vi "Start.vi"(8 "error in":errorcluster, 10 "ASync [T]":bool, 11 "ServiceBase out":refnum<class "ServiceBase.lvclass">) -> (0 "error out":errorcluster, 3 "ServiceBase out":refnum<class "ServiceBase.lvclass">)   [LabVIEW 2019, in "gRPC-servicer.lvlib" / "ServiceBase.lvclass"]
uses:
  ServiceBase.lvclass
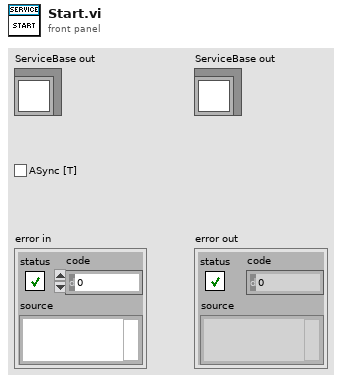
[diagram p1: front panel]
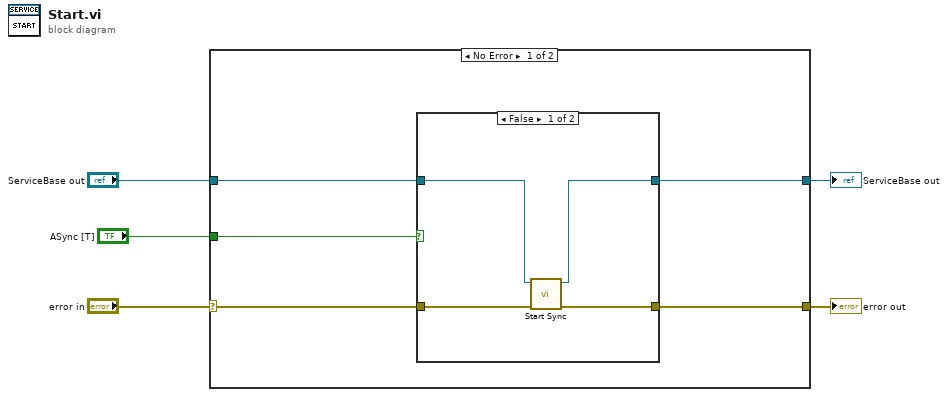
[diagram p0: block diagram]
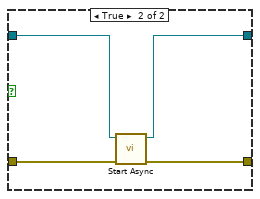
[diagram p2: hidden frame]
diagram:
  n1 = case shown="No Error" "error in" {
    selector: "error in" -> [w10 w20]
    tunnel: [w9 w20] -> w4
    tunnel: [w7 w19] -> w2
    tunnel: "ServiceBase out" -> [w8 w19]
    tunnel: "ASync [T]" -> [w6 _]
    frame No Error {
      n2 = case shown="False" w6 {
        tunnel: w10 -> [w14 w18]
        tunnel: [w13 w17] -> w9
        tunnel: w8 -> [w12 w16]
        tunnel: [w11 w15] -> w7
        frame False {
          n3 = call-dynamic "Start Sync.vi"("error in"=w14, "ServiceBase out"=w12) -> ("error out"=w13:errorcluster, "ServiceBase out"=w11:refnum<class "ServiceBase.lvclass">)  [unwired: 8 in]
        }
        frame True {
          n4 = call-dynamic "Start Async.vi"("error in"=w18, "ServiceBase in"=w16) -> ("error out"=w17:errorcluster, "ServiceBase out"=w15:refnum<class "ServiceBase.lvclass">)  [unwired: 8 in]
        }
      }
    }
    frame Error {
    }
  }
  "error out" <- w4
  "ServiceBase out" <- w2
